vi "Oracle DateTime to Labview TimeStamp.vi"(8 "error in":errorcluster, 11 "BD Date":string) -> (0 "error out":errorcluster, 3 "time stamp":timestamp)   [LabVIEW 2020, in "Oracle Driver.lvlib"]
uses:
  Oracle Driver.lvlib
  <vilib>/Utility/miscctls.llb/LVDateTimeRec.ctl
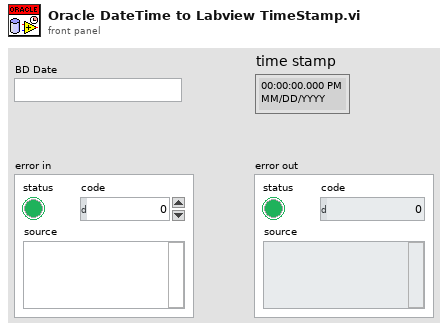
[diagram p1: front panel]
types:
  T1 = typedef "LVDateTimeRec.ctl" = cluster{"fractional second":dbl, "second":i32, "minute":i32, "hour":i32, "day of month":i32, "month":i32, "year":i32, "day of week":i32, "day of year":i32, "DST":i32}
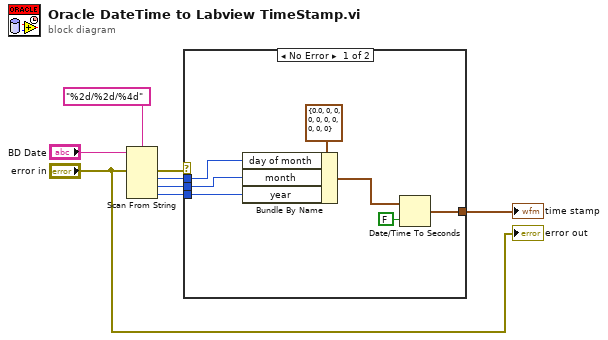
[diagram p0: block diagram]
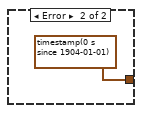
[diagram p2: hidden frame]
diagram:
  n1 = Scan From String(format string="%2d/%2d/%4d", input string="BD Date", error in="error in") -> (error out=w2:errorcluster, output 1=w6:i32, output 2=w5:i32, output 3=w4:i32)  [unwired: 4 in, 2 out]
  n2 = case shown="No Error" w2 {
    tunnel: w6 -> [w13 _]
    tunnel: w5 -> [w12 _]
    tunnel: w4 -> [w11 _]
    tunnel: [w10 timestamp(0 s since 1904-01-01) ("time stamp")] -> w3
    frame No Error {
      n3 = Bundle By Name(cluster=T1 {"fractional second"=0.0, "second"=0, "minute"=0, "hour"=0, "day of month"=0, "month"=0, "year"=0, "day of week"=0, "day of year"=0, "DST"=0} ("date time rec"), "day of month"=w13, "month"=w12, "year"=w11) -> (w15:T1)
      n4 = Date/Time To Seconds(1:FALSE ("is UTC (F)"), 2:w15) -> (0:w10:timestamp)
    }
    frame Error {
    }
  }
  "time stamp" <- w3
  "error out" <- "error in"
